vi "SysLogHistory Datei lesen PC.vi"(7 "History File":string, 8 "Fehler (in)":errorcluster caption="Fehlerkonstante") -> (0 "Fehler (out)":errorcluster caption="Fehlerkonstante", 3 "Array-Typ (2D Dbl)":string[][](array[string]))   [LabVIEW 2015, in "SysLog.lvlib"]
uses:
  SysLog.lvlib
  Allgemein/allgemeine Sub-VIs.lvlib
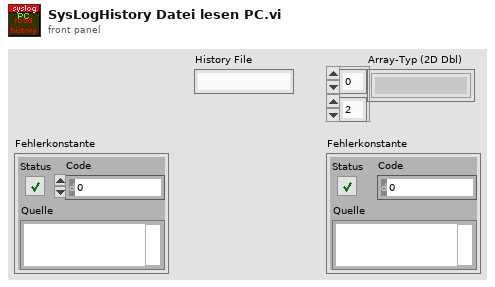
[diagram p1: front panel]
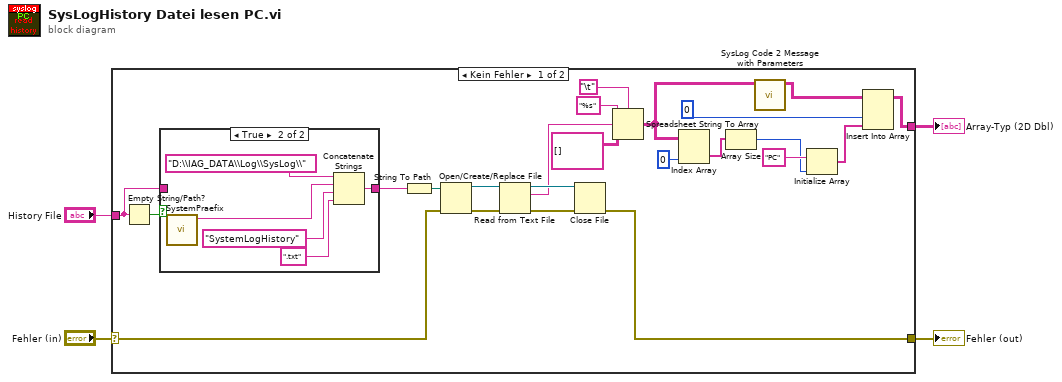
[diagram p0: block diagram]
diagram:
  n1 = case shown="Kein Fehler" "Fehler (in)" {
    selector: "Fehler (in)" -> [w10 w34]
    tunnel: [w9 w34] -> w3
    tunnel: [w21 _] -> w2
    tunnel: "History File" -> [w7 _]
    frame No Error {
      n2 = Empty String/Path?(string/path=w7) -> (empty?=w8:bool)
      n3 = case shown="True" w8 {
        tunnel: [w28 w31] -> w27
        tunnel: w7 -> [w28 _]
        frame False {
        }
        frame True {
          n4 = call "SystemPraefix.vi"() -> ("SystemPraefix"=w29:string)  [unwired: 10 in, 1 out]
          n5 = Concatenate Strings("D:\\IAG_DATA\\Log\\SysLog\\", w29, "SystemLogHistory" ("Dateiname"), ".txt" ("Dateiname")) -> (w31:string)
        }
      }
      n6 = String To Path(string=w27) -> (path=w17:path)
      n7 = Open/Create/Replace File(file path (use dialog)=w17, error in=w10) -> (refnum out=w26:refnum<file>, error out=w25:errorcluster)  [unwired: 4 in, 1 out]
      n8 = Read from Text File(file (use dialog)=w26, error in=w25) -> (refnum out=w24:refnum<file>, text=w15:string, error out=w23:errorcluster)  [unwired: 2 in, 1 out]
      n9 = Close File(refnum=w24, error in=w23) -> (error out=w9:errorcluster)  [unwired: 1 out]
      n10 = Spreadsheet String To Array(delimiter (Tab)="\t", format string="%s" ("Tabellen-String"), spreadsheet string=w15, array type (2D Dbl)=string[][] [] ("Array-Typ (2D Dbl)")) -> (array=w6:string[][])
      n11 = Index Array(array=w6, index (col)=0 ("Deaktivierter Index (Spalte)")) -> (element=w11:string[])  [unwired: 1 in]
      n12 = Array Size(array=w11) -> (size(s)=w13:i32)
      n13 = call "SysLog Code 2 Message with Parameters.vi"("Array-Typ (2D Dbl) (Eingang)"=w6) -> ("Array-Typ (2D Dbl) (Ausgang)"=w5:string[][])  [unwired: 10 in]
      n14 = Initialize Array("PC", w13) -> (w19:string[])
      n15 = Insert Into Array(array=w5, index (col)=0 ("Index (Zeile)"), new element=w19) -> (w21:string[][])  [unwired: 1 in]
    }
    frame Error {
    }
  }
  "Fehler (out)" <- w3
  "Array-Typ (2D Dbl)" <- w2
